vi "Initialize.vi"(8 "error in (no error)":errorcluster, 10 "CommandText":string, 11 "PathCommands in":refnum<class "PathCommands.lvclass">) -> (0 "error out":errorcluster, 3 "PathCommands out":refnum<class "PathCommands.lvclass">)   [LabVIEW 2019, in "PathCommands.lvclass"]
uses:
  PathCommands.lvclass
  <vilib>/Utility/error.llb/whitespace.ctl
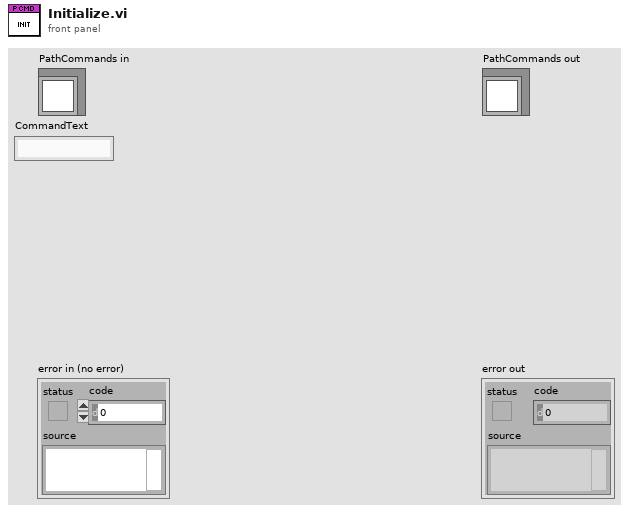
[diagram p1: front panel]
types:
  T1 = typedef "whitespace.ctl" = u16
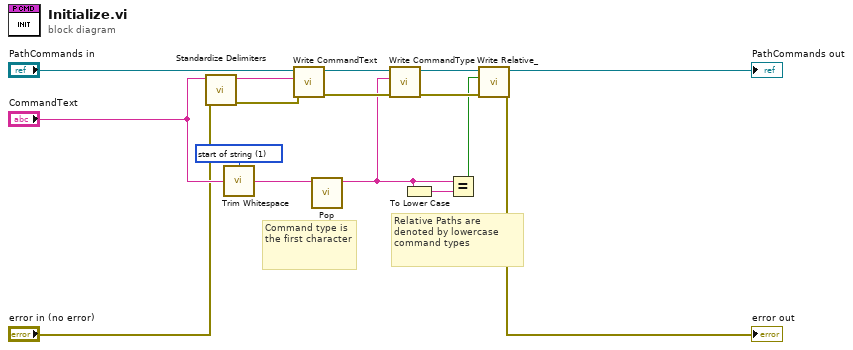
[diagram p0: block diagram]
diagram:
  w7 = T1 1 items=["both", "start of string", "end of string"] ("location (both)")
  # "Relative Paths are denoted by lowercase command types"
  # "Command type is the first character"
  n1 = call "Standardize Delimiters.vi"("error in (no error)"="error in (no error)", "Command In"="CommandText") -> ("error out"=w1:errorcluster, "Command Out"=w3:string)  [unwired: 8 in]
  n2 = call <vilib>:"Trim Whitespace.vi"("string"="CommandText", "location (both)"=w7) -> ("trimmed string"=w6:string)
  n3 = call-dynamic "Write CommandText.vi"("error in (no error)"=w1, "CommandText"=w3, "PathCommands in"="PathCommands in") -> ("error out"=w10:errorcluster, "PathCommands out"=w13:refnum<class "PathCommands.lvclass">)  [unwired: 7 in]
  n4 = call "Pop.vi"("Command Text"=w6) -> ("Command Type"=w5:string)  [unwired: 9 in, 1 out]
  n5 = call-dynamic "Write CommandType.vi"("error in (no error)"=w10, "CommandType"=w5, "PathCommands in"=w13) -> ("error out"=w11:errorcluster, "PathCommands out"=w12:refnum<class "PathCommands.lvclass">)  [unwired: 7 in]
  n6 = To Lower Case(string=w5) -> (all lower case string=w9:string)
  n7 = Equal?(x=w5, y=w9) -> (x = y?=w8:bool)
  n8 = call-dynamic "Write Relative_.vi"("error in (no error)"=w11, "Relative?"=w8, "PathCommands in"=w12) -> ("error out"=→"error out":errorcluster, "PathCommands out"=→"PathCommands out":refnum<class "PathCommands.lvclass">)  [unwired: 7 in]
